vi "SendMotorCmd.vi"(10 "Command Type":T1, 11 "Command Data":variant) -> ()   [LabVIEW 2011]
uses:
  Typedefs/CmdEnum_MotorIn.ctl
  Typedefs/Cmd_MotorIn.ctl
  GlobalVariables.vi
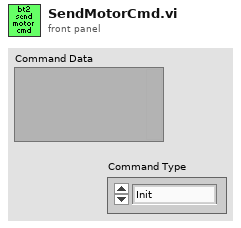
[diagram p1: front panel]
types:
  T1 = typedef "CmdEnum_MotorIn.ctl" = enum32{"Init", "Close", "SetPosition", "UpdatePositions", "MoveToLimit"}
  T2 = typedef "Cmd_MotorIn.ctl" = cluster{"Command Type":T1, "Msg Data":variant}
  T3 = typedef "QueueListType.ctl" = cluster{"Motor In":refnum<queue>, "User Interface Image View":refnum<queue>, "User Interface Camera Control":refnum<queue>, "User Interface Event Notifier":refnum<notifier>, "Initialized?":bool}
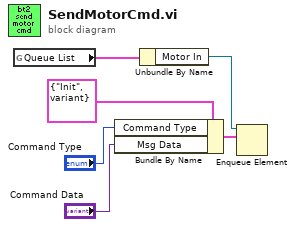
[diagram p0: block diagram]
diagram:
  n1 = global read "GlobalVariables.vi" "Queue List"() -> (w6:T3)
  n2 = Bundle By Name(cluster=T2 {"Command Type"=enum."Init", "Msg Data"=variant} ("Cluster"), "Command Type"="Command Type", "Msg Data"="Command Data") -> (w1:T2)
  n3 = Unbundle By Name(w6) -> ("Motor In"=w5:refnum<queue>)
  n4 = Enqueue Element(queue=w5, element=w1) -> ()  [unwired: 2 in, 3 out]
